vi "save dataset.vi"(9 "old dataset":T2, 10 "X-wave column":i8=-1, 11 "Y-wave columns":u8[](array[numeric])=[1]) -> (1 "new dataset":T2)   [LabVIEW 2025]
panel:
  in  "Save Mode":T1(ring)
  in  "Done":bool
  in  "Cancel button":bool
  # "Save the data files into a packaged data format."
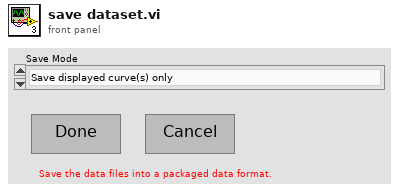
[diagram p1: front panel]
types:
  T1 = enum16{"Save displayed curve(s) only", "Save the whole datasets with displayed curve(s)", "Save the whole datasets regardless of the curves displayed", "Save into two seprate files with displayed and undisplayed curves each"}
  T2 = cluster{"data cluster":cluster{"all data":dbl[][]}[], "Scale":u16, "scale matrix":dbl[][], "universal y-scale":dbl, "data names":string[], "new dataset?":bool, "show files 2":cluster{"String":string, "Boolean":bool, "begin":u32, "length":u32, "y weight":dbl}[]}
  T3 = enum16{"open", "replace", "create", "open or create", "replace or create", "replace or create with confirmation"}
  T4 = cluster{"String":string, "Boolean":bool, "begin":u32, "length":u32, "y weight":dbl}[]
  T5 = cluster{cluster{"all data":dbl[][]}[], "Scale":u16, "scale matrix":dbl[][], "universal y-scale":dbl, string[], "new dataset?":bool, cluster{"String":string, "Boolean":bool, "begin":u32, "length":u32, "y weight":dbl}[]}
  T6 = cluster{cluster{dbl[][]}[], "Scale":u16, "scale matrix":dbl[][], "universal y-scale":dbl, string[], "new dataset?":bool, cluster{"String":string, "Boolean":bool, "begin":u32, "length":u32, "y weight":dbl}[]}
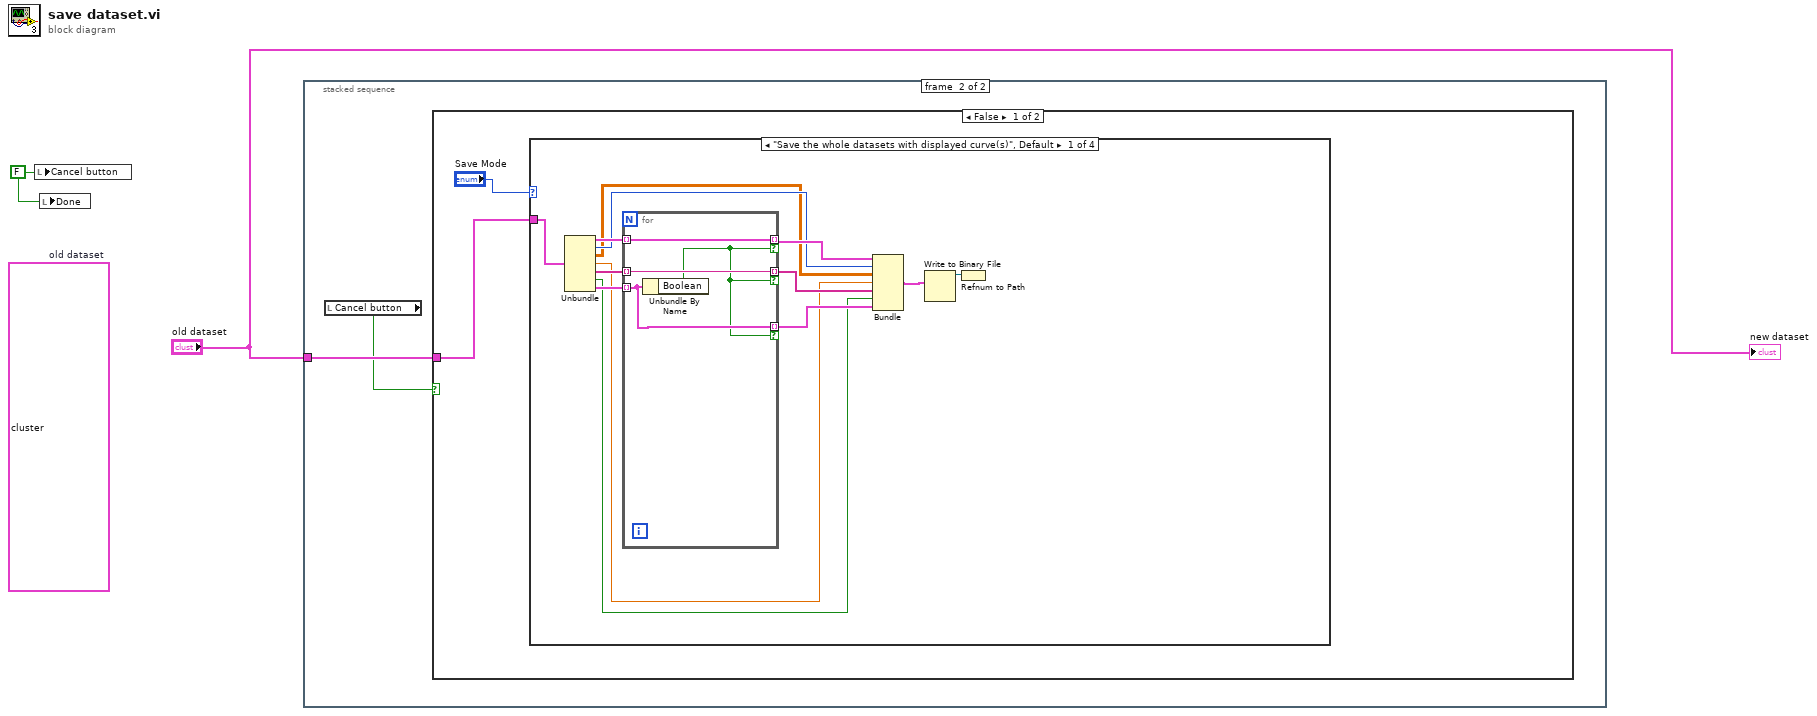
[diagram p0: block diagram]
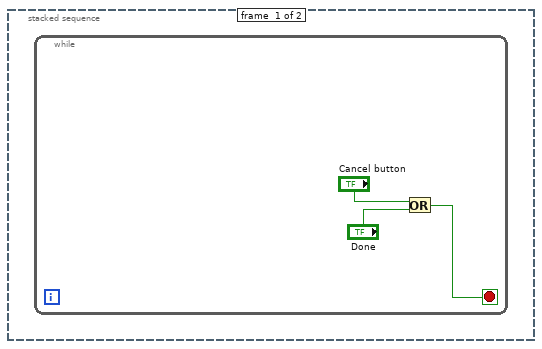
[diagram p2: hidden frame]
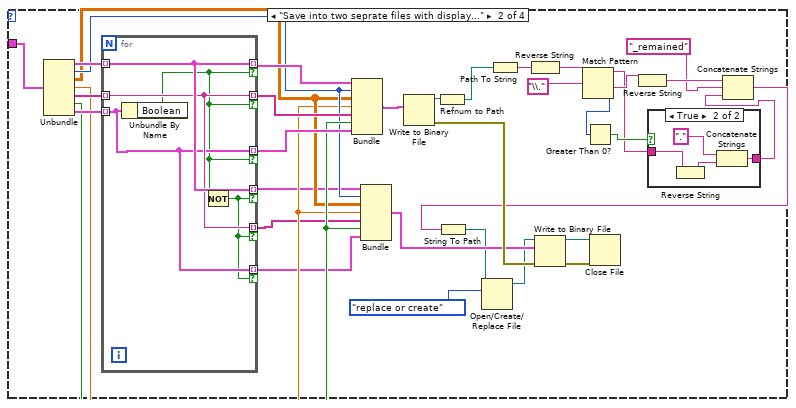
[diagram p3: hidden frame]
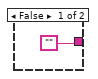
[diagram p4: hidden frame]
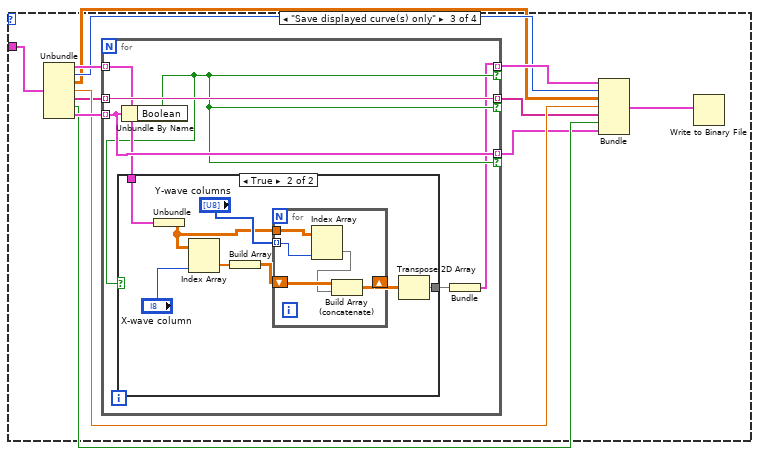
[diagram p5: hidden frame]
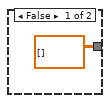
[diagram p6: hidden frame]
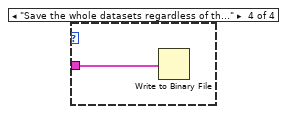
[diagram p7: hidden frame]
diagram:
  w1 = FALSE ("Cancel button")
  (unwired) T2 {"data cluster"=[{"all data"=array60x36[2160 elements]}], "Scale"=0, "scale matrix"=[], "universal y-scale"=1.0, "data names"=["FGT512para_PPMS_Hsweep_170K3.dat"], "new dataset?"=TRUE, "show files 2"=[]}  # old dataset
  n1 = local write "Cancel button"(w1) -> ()
  n2 = local write "Done"(w1) -> ()
  n3 = stacked-sequence {
    tunnel: "old dataset" -> [_ w7]
    frame #0 {
      n4 = while {
        stop <- w3 stop-if-true
        n5 = Or(x="Cancel button", y="Done") -> (x .or. y?=w3:bool)
      }
    }
    frame #1 {
      n6 = local read "Cancel button"() -> (w6:bool)
      n7 = case shown="False" w6 {
        tunnel: w7 -> [w9 _]
        frame False {
          n8 = case shown="\"Save the whole datasets with displayed curve(s)\", Default" "Save Mode" {
            tunnel: w9 -> [w20 w59 w81 w104]
            frame "Save the whole datasets with displayed curve(s)", Default {
              n9 = Unbundle(w20) -> ("data cluster"=w21:cluster{"all data":dbl[][]}[], "Scale"=w14:u16, "scale matrix"=w13:dbl[][], "universal y-scale"=w12:dbl, "data names"=w18:string[], "new dataset?"=w15:bool, "show files 2"=w22:T4)
              n10 = for {
                tunnel: w22 -> [w24] mode=indexing
                tunnel: w21 -> [w26] mode=indexing
                tunnel: [w26] -> w19 mode=indexing if=w23
                tunnel: w18 -> [w25] mode=indexing
                tunnel: [w25] -> w17 mode=indexing if=w23
                tunnel: [w24] -> w16 mode=indexing if=w23
                n11 = Unbundle By Name(w24) -> ("Boolean"=w23:bool)
              }
              n12 = Bundle(w19, "Scale"=w14, "scale matrix"=w13, "universal y-scale"=w12, w17, "new dataset?"=w15, w16) -> (w11:T5)  [unwired: 1 in]
              n13 = Write to Binary File(data=w11) -> (refnum out=w10:refnum<file>)  [unwired: 5 in, 2 out]
              n14 = Refnum to Path(1:w10) -> ()  [unwired: 1 out]
            }
            frame "Save into two seprate files with displayed and undisplayed curves each" {
              n15 = Unbundle(w59) -> ("data cluster"=w60:cluster{"all data":dbl[][]}[], "Scale"=w53:u16, "scale matrix"=w52:dbl[][], "universal y-scale"=w51:dbl, "data names"=w57:string[], "new dataset?"=w54:bool, "show files 2"=w61:T4)
              n16 = for {
                tunnel: w61 -> [w69] mode=indexing
                tunnel: w60 -> [w71] mode=indexing
                tunnel: [w71] -> w58 mode=indexing if=w68
                tunnel: w57 -> [w70] mode=indexing
                tunnel: [w70] -> w56 mode=indexing if=w68
                tunnel: [w69] -> w55 mode=indexing if=w68
                tunnel: [w71] -> w50 mode=indexing if=w67
                tunnel: [w70] -> w49 mode=indexing if=w67
                tunnel: [w69] -> w48 mode=indexing if=w67
                n17 = Unbundle By Name(w69) -> ("Boolean"=w68:bool)
                n18 = Not(x=w68) -> (.not. x?=w67:bool)
              }
              n19 = Bundle(w58, "Scale"=w53, "scale matrix"=w52, "universal y-scale"=w51, w56, "new dataset?"=w54, w55) -> (w47:T5)  [unwired: 1 in]
              n20 = Bundle(w50, "Scale"=w53, "scale matrix"=w52, "universal y-scale"=w51, w49, "new dataset?"=w54, w48) -> (w44:T5)  [unwired: 1 in]
              n21 = Write to Binary File(data=w47) -> (refnum out=w46:refnum<file>, error out=w45:errorcluster)  [unwired: 5 in, 1 out]
              n22 = Refnum to Path(1:w46) -> (0:w40:path)
              n23 = Path To String(path=w40) -> (string=w39:string)
              n24 = Reverse String(1:w39) -> (0:w38:string)
              n25 = Match Pattern(string=w38, regular expression="\\.") -> (before substring=w32:string, after substring=w37:string, offset past match=w33:i32)  [unwired: 1 in, 1 out]
              n26 = Greater Than 0?(x=w33) -> (x > 0?=w34:bool)
              n27 = Reverse String(1:w37) -> (0:w36:string)
              n28 = case shown="True" w34 {
                tunnel: w32 -> [_ w66]
                tunnel: ["" w65] -> w29
                frame False {
                }
                frame True {
                  n29 = Reverse String(1:w66) -> (0:w64:string)
                  n30 = Concatenate Strings("." ("string"), w64) -> (w65:string)
                }
              }
              n31 = Concatenate Strings(w36, "_remained", w29) -> (w30:string)
              n32 = String To Path(string=w30) -> (path=w27:path)
              n33 = Open/Create/Replace File(file path (use dialog)=w27, operation (0:open)=T3."replace or create") -> (refnum out=w43:refnum<file>)  [unwired: 4 in, 2 out]
              n34 = Write to Binary File(file (use dialog)=w43, data=w44, error in=w45) -> (refnum out=w28:refnum<file>, error out=w41:errorcluster)  [unwired: 3 in, 1 out]
              n35 = Close File(refnum=w28, error in=w41) -> ()  [unwired: 2 out]
            }
            frame "Save displayed curve(s) only" {
              n36 = Unbundle(w81) -> ("data cluster"=w82:cluster{"all data":dbl[][]}[], "Scale"=w79:u16, "scale matrix"=w78:dbl[][], "universal y-scale"=w77:dbl, "data names"=w76:string[], "new dataset?"=w74:bool, "show files 2"=w83:T4)
              n37 = for {
                tunnel: w83 -> [w88] mode=indexing
                tunnel: w82 -> [w87] mode=indexing
                tunnel: [w84] -> w80 mode=indexing if=w86
                tunnel: w76 -> [w89] mode=indexing
                tunnel: [w89] -> w75 mode=indexing if=w86
                tunnel: [w88] -> w73 mode=indexing if=w86
                n38 = Unbundle By Name(w88) -> ("Boolean"=w86:bool)
                n39 = case shown="True" w86 {
                  tunnel: w87 -> [_ w98]
                  tunnel: [dbl[][] [] w91] -> w85
                  frame False {
                  }
                  frame True {
                    n40 = Unbundle(w98) -> ("all data"=w95:dbl[][])
                    n41 = Index Array(array=w95, index (col)="X-wave column") -> (element=w94:dbl[])  [unwired: 1 in]
                    n42 = Build Array(w94) -> (w93:dbl[][])
                    n43 = for {
                      tunnel: "Y-wave columns" -> [w102] mode=indexing
                      tunnel: w95 -> [w103]
                      shift-right: [w99] -> w92
                      shift-left: w93 -> [w101]
                      n44 = Index Array(array=w103, index (col)=w102) -> (element=w100:dbl[])  [unwired: 1 in]
                      n45 = Build Array (concatenate)(w101, w100) -> (w99:dbl[][])
                    }
                    n46 = Transpose 2D Array(2D array=w92) -> (transposed array=w91:dbl[][])
                  }
                }
                n47 = Bundle(w85) -> (w84:cluster{dbl[][]})  [unwired: 1 in]
              }
              n48 = Bundle(w80, "Scale"=w79, "scale matrix"=w78, "universal y-scale"=w77, w75, "new dataset?"=w74, w73) -> (w72:T6)  [unwired: 1 in]
              n49 = Write to Binary File(data=w72) -> ()  [unwired: 5 in, 3 out]
            }
            frame "Save the whole datasets regardless of the curves displayed" {
              n50 = Write to Binary File(data=w104) -> ()  [unwired: 5 in, 3 out]
            }
          }
        }
        frame True {
        }
      }
    }
  }
  "new dataset" <- "old dataset"
